vi "Add Value Column.vi"(11 "Series in":refnum<class "Series.lvclass">) -> (3 "Series out":refnum<class "Series.lvclass">)   [LabVIEW 2018, in "InfluxDB Client.lvlib" / "Series.lvclass"]
uses:
  Series.lvclass
  Series.lvclass/Series.ctl
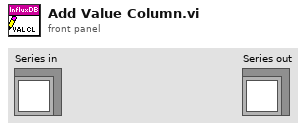
[diagram p1: front panel]
types:
  T1 = typedef "Dictionary Object RefNum__ogtk.ctl" = refnum<k1>
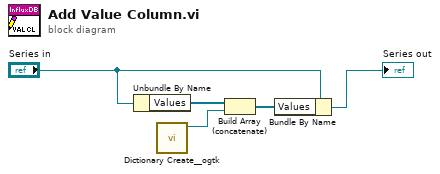
[diagram p0: block diagram]
diagram:
  n1 = Unbundle By Name("Series in") -> ("Values"=w3:T1[])
  n2 = call <userlib>:"Dictionary Create__ogtk.vi"() -> ("dictionary out"=w1:T1)  [unwired: 10 in, 1 out]
  n3 = Build Array (concatenate)(w3, w1) -> (w2:T1[])
  n4 = Bundle By Name(cluster="Series in", "Values"=w2) -> (→"Series out":refnum<class "Series.lvclass">)
